vi "sweep_finished.vi"(8 "error in (no error)":errorcluster, 11 "DataCollectionDL110128Streaming in":refnum<class "DataCollectionDL110128Streaming.lvclass">) -> (0 "error out":errorcluster, 3 "DataCollectionDL110128Streaming out":refnum<class "DataCollectionDL110128Streaming.lvclass">)   [LabVIEW 2010, in "DataCollectionDL110128Streaming.lvclass"]
uses:
  DataCollectionDL110128Streaming.lvclass
  DataCollectionDL110128Streaming.lvclass/DataCollectionDL110128Streaming.ctl
  GenericDataCollection/GenericDataCollection/trigger_enum.ctl
  GenericDataCollection/GenericDataCollection/GenericDataCollection.lvclass
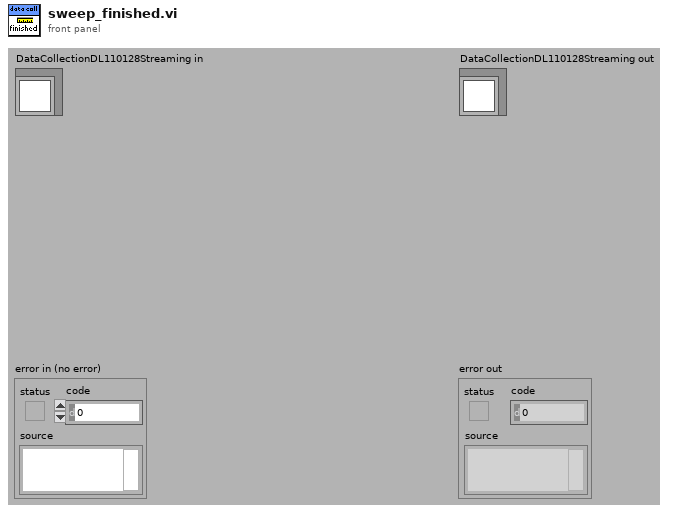
[diagram p1: front panel]
types:
  T1 = typedef "GenericDataCollection.lvclass/trigger_enum.ctl" = enum16{"NULL", "save", "reset"}
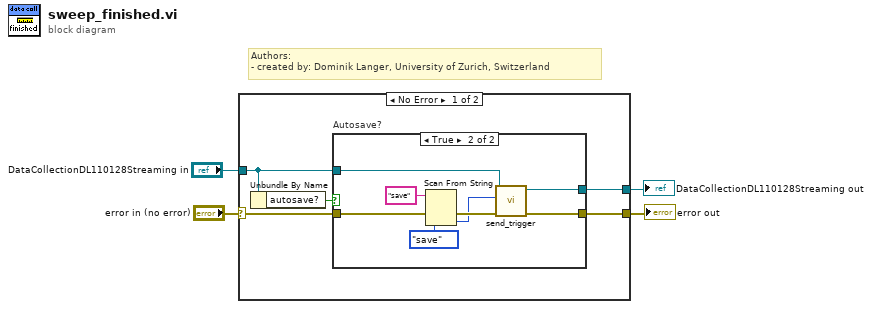
[diagram p0: block diagram]
diagram:
  # "Authors: \n- created by: Dominik Langer, University of Zurich, Switzerland"
  n1 = case shown="No Error" "error in (no error)" {
    selector: "error in (no error)" -> [w9 w20]
    tunnel: "DataCollectionDL110128Streaming in" -> [w6 w21]
    tunnel: [w7 w20] -> w2
    tunnel: [w5 w21] -> w1
    frame No Error {
      n2 = Unbundle By Name(w6) -> ("autosave?"=w8:bool)
      n3 = case "Autosave?" shown="True" w8 {
        tunnel: w9 -> [w11 w18]
        tunnel: [w11 w16] -> w7
        tunnel: w6 -> [w10 w14]
        tunnel: [w10 w13] -> w5
        frame False {
        }
        frame True {
          n4 = Scan From String(input string="save", error in=w18, default 1=trigger_enum."save" ("trigger")) -> (error out=w17:errorcluster, output 1=w15:T1)  [unwired: 2 in, 2 out]
          n5 = call-dynamic "send_trigger.vi"("error in (no error)"=w17, "trigger"=w15, "GenericDataCollection in"=w14) -> ("error out"=w16:errorcluster, "GenericDataCollection out"=w13:refnum<class "DataCollectionDL110128Streaming.lvclass">)  [unwired: 7 in]
        }
      }
    }
    frame Error {
    }
  }
  "error out" <- w2
  "DataCollectionDL110128Streaming out" <- w1
